vi "SearchAndReplaceJit.vi"(4 "continue capture index":i32, 5 "replace capture index":i32, 6 "offset":i32, 7 "replace all (F)":bool, 8 "error in":errorcluster, 9 "replace to":string, 10 "search pattern":string, 11 "string":string) -> (0 "error out":errorcluster, 1 "offset past replacement":i32, 2 "number of replacements":i32, 3 "result string":string)   [LabVIEW 2021, in "libpcre2-8.lvlib"]
uses:
  libpcre2-8.lvlib
  Pcre2MoOfSubstrNumFmOv.vi
  Pcre2CompileError.vi
  Pcre2FnkCallError.vi
  Pcre2ErrorNull.vi
  Pcre2LibError.vi
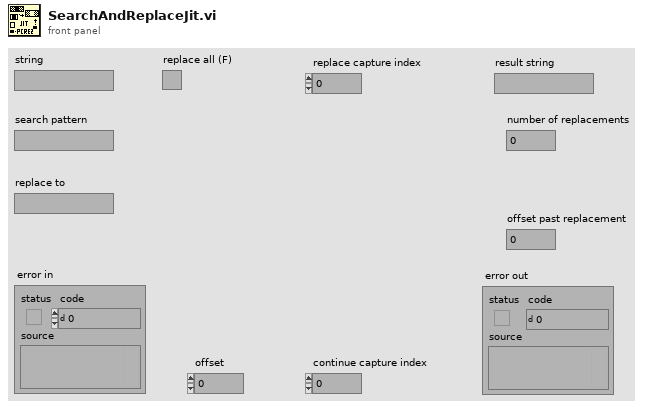
[diagram p1: front panel]
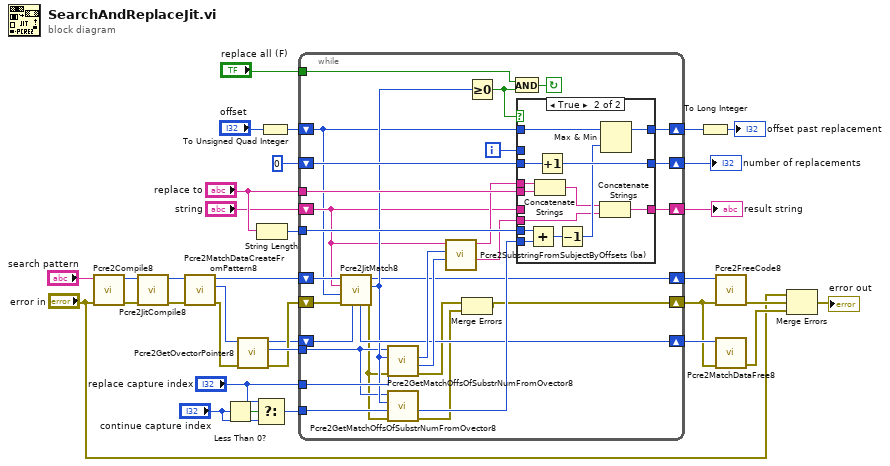
[diagram p0: block diagram]
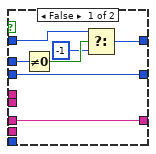
[diagram p2: hidden frame]
diagram:
  n1 = call "Pcre2Compile8.vi"("error in"="error in", "Pattern"="search pattern") -> ("error out"=w29:errorcluster, "pCode"=w26:u64)  [unwired: 8 in]
  n2 = call "Pcre2JitCompile8.vi"("error in"=w29, "pCode"=w26) -> ("error out"=w28:errorcluster, "pCode"=w25:u64)  [unwired: 8 in]
  n3 = call "Pcre2MatchDataCreateFromPattern8.vi"("error in"=w28, "pCode"=w25) -> ("error out"=w20:errorcluster, "pMatchData"=w22:u64, "pCode"=w24:u64)  [unwired: 7 in]
  n4 = Less Than 0?(x="continue capture index") -> (x < 0?=w32:bool)
  n5 = call "Pcre2GetOvectorPointer8.vi"("error in"=w20, "pMatchData"=w22) -> ("error out"=w19:errorcluster, "pOvector"=w21:u64, "pMatchData"=w18:u64)  [unwired: 7 in]
  n6 = Select(t="replace capture index", s=w32, f="continue capture index") -> (s? t:f=w33:i32)
  n7 = String Length(string="replace to") -> (length=w31:i32)
  n8 = To Unsigned Quad Integer(1:"offset") -> (0:w23:u64)
  n9 = while {
    shift-right: [w41] -> w16
    shift-left: w24 -> [w53]
    shift-right: [w34] -> w15
    shift-left: w19 -> [w52]
    shift-right: [w60] -> w10
    shift-left: w23 -> [w37]
    shift-right: [w62] -> w11
    shift-left: "string" -> [w38]
    shift-right: [w57] -> w9
    shift-left: 0 -> [w58]
    tunnel: "replace all (F)" -> [w56]
    tunnel: "replace to" -> [w55]
    tunnel: w31 -> [w54]
    tunnel: w33 -> [w45]
    tunnel: w21 -> [w40]
    tunnel: "replace capture index" -> [w50]
    shift-right: [w43] -> w17
    shift-left: w18 -> [w51]
    i -> [w59]
    stop <- w63 continue-if-true
    n10 = call "Pcre2JitMatch8.vi"("pMatchData"=w51, "error in"=w52, "StartOffset"=w37, "Subject"=w38, "pCode"=w53) -> ("error out"=w39:errorcluster, "MatchResult"=w42:i32, "pCode"=w41:u64, "pMatchData"=w43:u64)  [unwired: 3 in]
    n11 = call "Pcre2GetMatchOffsOfSubstrNumFromOvector8.vi"("error in"=w39, "Number"=w50, "MatchResult"=w42, "pOvector"=w40) -> ("error out"=w36:errorcluster, "OffsetPastMatch"=w48:i32, "MatchOffset"=w49:i32)  [unwired: 4 in, 1 out]
    n12 = call "Pcre2GetMatchOffsOfSubstrNumFromOvector8.vi"("error in"=w39, "Number"=w45, "MatchResult"=w42, "pOvector"=w40) -> ("error out"=w35:errorcluster, "OffsetPastMatch"=w44:i32)  [unwired: 4 in, 2 out]
    n13 = call "Pcre2SubstringFromSubjectByOffsets (ba).vi"("OffsetPastMatch"=w48, "MatchOffset"=w49, "Subject"=w38) -> ("AfterSubstring"=w46:string, "BeforeSubstring"=w47:string)  [unwired: 7 in]
    n14 = Merge Errors(w36, w35) -> (w34:errorcluster)
    n15 = Greater Or Equal To 0?(x=w42) -> (x >= 0?=w61:bool)
    n16 = And(x=w56, y=w61) -> (x .and. y?=w63:bool)
    n17 = case shown="True" w61 {
      tunnel: w47 -> [_ w83]
      tunnel: w46 -> [_ w71]
      tunnel: [w70 w82] -> w62
      tunnel: w38 -> [w70 _]
      tunnel: [w69 w78] -> w60
      tunnel: w59 -> [w67 _]
      tunnel: w37 -> [w66 w79]
      tunnel: w58 -> [w64 w81]
      tunnel: [w64 w80] -> w57
      tunnel: w55 -> [_ w77]
      tunnel: w44 -> [_ w74]
      tunnel: w54 -> [_ w76]
      frame False {
        n18 = Not Equal To 0?(x=w67) -> (x != 0?=w68:bool)
        n19 = Select(t=w66, s=w68, f=-1) -> (s? t:f=w69:u64)
      }
      frame True {
        n20 = Add(x=w76, y=w74) -> (x+y=w75:i32)
        n21 = Concatenate Strings(w83, w77) -> (w72:string)
        n22 = Increment(x=w81) -> (x+1=w80:i32)
        n23 = Decrement(x=w75) -> (x-1=w73:i32)
        n24 = Concatenate Strings(w72, w71) -> (w82:string)
        n25 = Max & Min(x=w79, y=w73) -> (max(x,y)=w78:u64)  [unwired: 1 out]
      }
    }
  }
  "result string" <- w11
  "number of replacements" <- w9
  n26 = To Long Integer(number=w10) -> (32bit integer=→"offset past replacement":i32)
  n27 = call "Pcre2FreeCode8.vi"("error in"=w15, "pCode"=w16) -> ("error out"=w14:errorcluster)  [unwired: 9 in]
  n28 = call "Pcre2MatchDataFree8.vi"("error in"=w15, "pMatchData"=w17) -> ("error out"=w3:errorcluster)  [unwired: 9 in]
  n29 = Merge Errors("error in", w14, w3) -> (→"error out":errorcluster)
